vi "BothSlopes_thread.vi"(1 "board":u32) -> ()   [LabVIEW 2015]
uses:
  lv64_eventdriven/board.vis/ESLSCDLL.dll
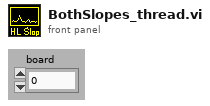
[diagram p1: front panel]
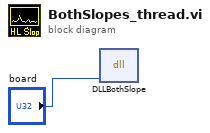
[diagram p0: block diagram]
diagram:
  n1 = dll-call lib="C:/ENTW/PCIE/64bit/lv64/lv64_eventdriven/board.vis/ESLSCDLL.dll" fn="DLLBothSlope" ("lwlscdll.dll:DLLHighSlope")("drv"="board") -> ()  [unwired: 5 in, 2 out]
